vi "Cannon Modifications.vi"(1 "Cannon Global Data In":T2) -> (0 "Cannon Global Data Out":T2)   [LabVIEW 2013]
uses:
  <vilib>/Rock Robotics/WPI/Solenoid/WPI_SolenoidValue.ctl
  InTake/InTake Global Data.vi
panel:
  in  "min intake angle to shoot":dbl format="%#_13g"
  in  "min cannon angle to shoot":dbl format="%#_13g"
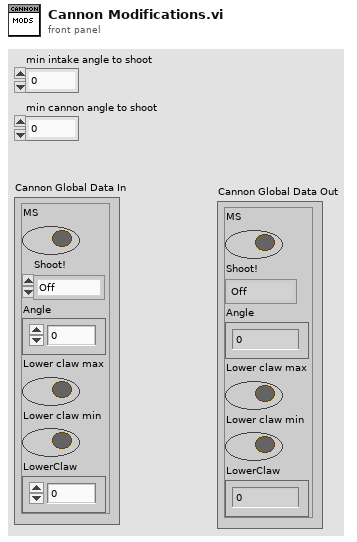
[diagram p1: front panel]
types:
  T1 = typedef "WPI_SolenoidValue.ctl" = enum16{"Off", "On", "Forward", "Reverse"}
  T2 = cluster{"MS":bool, "Shoot!":T1, "Angle":dbl, "Lower claw max":bool, "Lower claw min":bool, "LowerClaw":dbl}
  T3 = cluster{"TakeBall":dbl, "UpperClaw":dbl, "MS":bool, "Upper claw max":bool, "Upper claw min":bool, "Angle":dbl}
  T4 = typedef "WPI_GyroDevRef.ctl" = cluster{"DevStatus":errorcluster, "Analog Module":T5, "Analog Channel":T6, "Offset":dbl, "Gain (VoltsPerDegree/Second)":dbl}
  T5 = typedef "FPGA_TypedefAnalogModule.ctl" = enum16{"Analog Module 1", "Analog Module 2"}
  T6 = typedef "FPGA_AIChannel.ctl" = enum8{"AI 1", "AI 2", "AI 3", "AI 4", "AI 5", "AI 6", "AI 7", "AI 8", "Invalid"}
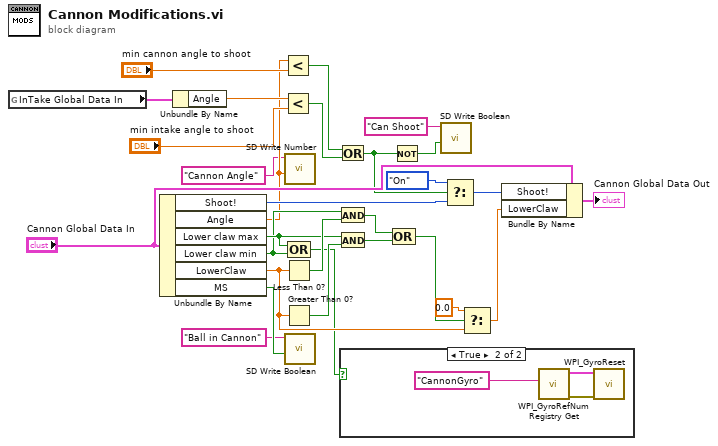
[diagram p0: block diagram]
diagram:
  n1 = global read "InTake Global Data.vi" "InTake Global Data In"() -> (w12:T3)
  n2 = Unbundle By Name("Cannon Global Data In") -> ("Shoot!"=w13:T1, "Angle"=w4:dbl, "Lower claw max"=w17:bool, "Lower claw min"=w16:bool, "LowerClaw"=w19:dbl, "MS"=w2:bool)
  n3 = Unbundle By Name(w12) -> ("Angle"=w9:dbl)
  n4 = Less?(x=w4, y="min cannon angle to shoot") -> (x < y?=w11:bool)
  n5 = Less?(x=w9, y="min intake angle to shoot") -> (x < y?=w10:bool)
  n6 = Less Than 0?(x=w19) -> (x < 0?=w21:bool)
  n7 = Greater Than 0?(x=w19) -> (x > 0?=w22:bool)
  n8 = call <vilib>:"SD Write Number.vi"("Numeric"=w4, "Name"="Cannon Angle") -> ()  [unwired: 8 in, 2 out]
  n9 = call <vilib>:"SD Write Boolean.vi"("Boolean"=w2, "Name"="Ball in Cannon") -> ()  [unwired: 8 in, 2 out]
  n10 = Compound Arithmetic op=OR(w17, w16) -> (w15:bool)
  n11 = Or(x=w11, y=w10) -> (x .or. y?=w7:bool)
  n12 = And(x=w16, y=w21) -> (x .and. y?=w23:bool)
  n13 = And(x=w17, y=w22) -> (x .and. y?=w24:bool)
  n14 = case shown="True" w15 {
    frame False {
    }
    frame True {
      n15 = call <vilib>:"WPI_GyroRefNum Registry Get.vi"("refnum name"="CannonGyro") -> ("error out"=w31:errorcluster, "GyroDevRef"=w30:T4)  [unwired: 9 in]
      n16 = call <vilib>:"WPI_GyroReset.vi"("error in (no error)"=w31, "GyroDevRef"=w30) -> ()  [unwired: 8 in, 2 out]
    }
  }
  n17 = Not(x=w7) -> (.not. x?=w6:bool)
  n18 = Compound Arithmetic op=OR(w23, w24) -> (w25:bool)
  n19 = call <vilib>:"SD Write Boolean.vi"("Boolean"=w6, "Name"="Can Shoot") -> ()  [unwired: 8 in, 2 out]
  n20 = Select(t=WPI_SolenoidValue."On" ("Shoot!"), s=w7, f=w13) -> (s? t:f=w27:T1)
  n21 = Select(t=0.0, s=w25, f=w19) -> (s? t:f=w18:dbl)
  n22 = Bundle By Name(cluster="Cannon Global Data In", "Shoot!"=w27, "LowerClaw"=w18) -> (→"Cannon Global Data Out":T2)
